vi "VS Errors_Display and Log Custom Device Error.vi"(8 "error out":errorcluster, 9 "Note (empty)":string, 10 "Your code's public name":string, 11 "Custom Device? (T)":bool=TRUE) -> ()   [LabVIEW 2013, in "CANOpen Addon Custom Device.lvlib"]
uses:
  CANOpen Addon Custom Device.lvlib
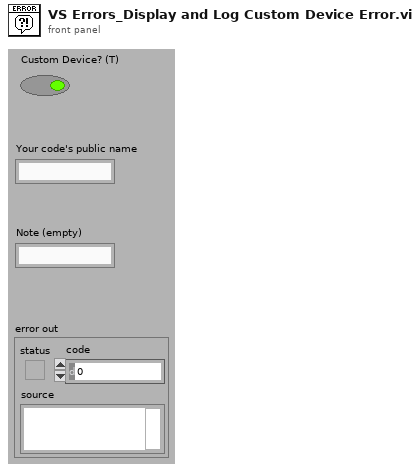
[diagram p1: front panel]
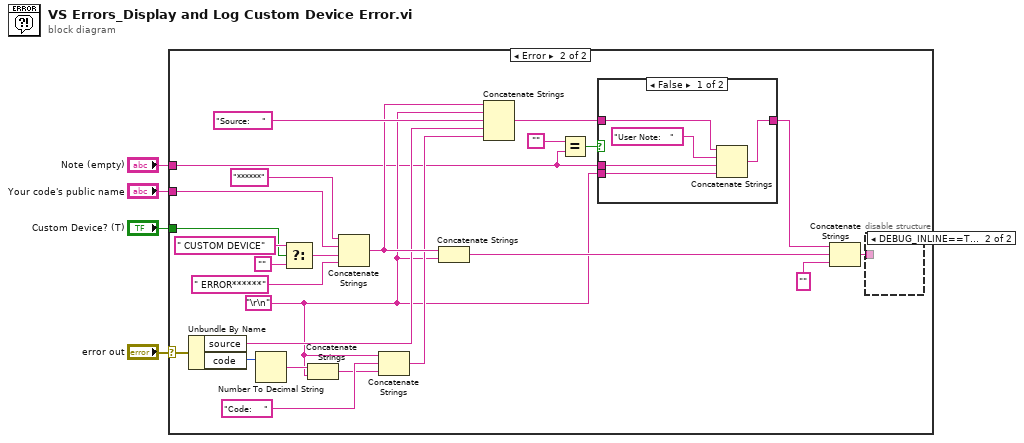
[diagram p0: block diagram]
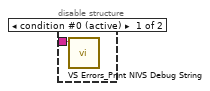
[diagram p3: hidden frame]
diagram:
  n1 = case shown="Error" "error out" {
    selector: "error out" -> [_ w29]
    tunnel: "Custom Device? (T)" -> [_ w17]
    tunnel: "Your code's public name" -> [_ w7]
    tunnel: "Note (empty)" -> [_ w5]
    frame No Error {
    }
    frame Error {
      w6 = "\r\n"
      n2 = Unbundle By Name(w29) -> ("source"=w16:string, "code"=w9:i32)
      n3 = Number To Decimal String(number=w9) -> (decimal integer string=w26:string)  [unwired: 1 in]
      n4 = Select(t=" CUSTOM DEVICE" ("String"), s=w17, f="") -> (s? t:f=w18:string)
      n5 = Concatenate Strings(w26, w6) -> (w8:string)
      n6 = Concatenate Strings("******" ("String"), w7, w18, " ERROR******" ("String")) -> (w21:string)
      n7 = Concatenate Strings(w6, "Code:    " ("String"), w8) -> (w15:string)
      n8 = Concatenate Strings(w21, w6) -> (w12:string)
      n9 = Concatenate Strings(w21, w6, "Source:    " ("String"), w16, w15) -> (w14:string)
      n10 = Equal?(x="", y=w5) -> (x = y?=w19:bool)
      n11 = case shown="False" w19 {
        tunnel: w5 -> [w34 _]
        tunnel: w6 -> [w33 _]
        tunnel: w14 -> [w32 w36]
        tunnel: [w31 w36] -> w13
        frame False {
          n12 = Concatenate Strings(w32, "User Note:   " ("string"), w34, w33) -> (w31:string)
        }
        frame True {
        }
      }
      n13 = Concatenate Strings(w13, w12, "" ("Message")) -> (w10:string)
      n14 = disable-structure shown="DEBUG_INLINE==TRUE" {
        disable-tunnel: w10 -> [w30 _]
        frame condition #0 (active) {
          n15 = call "VS Errors_Print NIVS Debug String.vi"("Debug String"=w30) -> ()  [unwired: 9 in, 1 out]
        }
        frame condition #1 {
        }
      }
    }
  }
